vi "Maximize.vi"(8 "error in":errorcluster, 11 "Flex Subpanel in":refnum<class "Flex UI Subpanel.lvclass">) -> (0 "error out":errorcluster, 3 "Flex Subpanel out":refnum<class "Flex UI Subpanel.lvclass">)   [LabVIEW 2016, in "Flex UI Subpanel.lvclass"]
doc: "Maximizes the UI."
uses:
  Flex UI Subpanel.lvclass
  <vilib>/Utility/miscctls.llb/LVPositionTypeDef.ctl
  Flex UI Subpanel.lvclass/Flex UI Subpanel.ctl
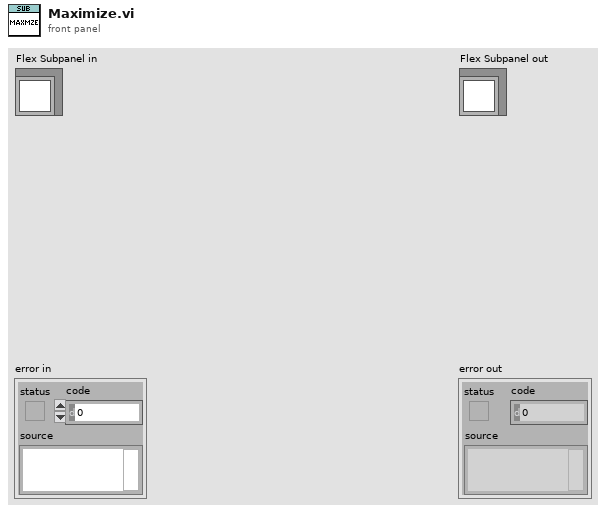
[diagram p1: front panel]
types:
  T1 = typedef "LVPositionTypeDef.ctl" = cluster{"Left":i32, "Top":i32}
  T2 = typedef "LVBoundsTypeDef.ctl" = cluster{"Width":u32, "Height":u32}
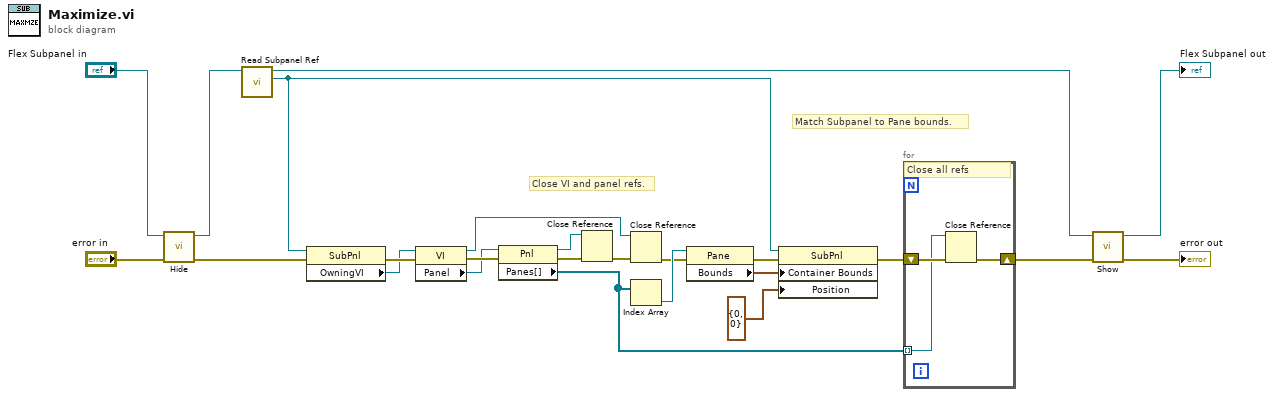
[diagram p0: block diagram]
diagram:
  # "Match Subpanel to Pane bounds."
  # "Close VI and panel refs."
  n1 = call-dynamic "Hide.vi"("error in"="error in", "Flex Subpanel in"="Flex Subpanel in") -> ("error out"=w4:errorcluster, "Flex Subpanel out"=w2:refnum<class "Flex UI Subpanel.lvclass">)  [unwired: 8 in]
  n2 = call "Read Subpanel Ref.vi"("Flex Subpanel in"=w2) -> ("Subpanel Ref"=w12:refnum<vi>, "Flex Subpanel out"=w20:refnum<class "Flex UI Subpanel.lvclass">)  [unwired: 9 in]
  n3 = property class="SubPnl"(reference=w12, error in=w4) -> (error out=w22:errorcluster, "OwningVI"=w18:refnum<vi>)  [unwired: 1 out]
  n4 = property class="VI"(reference=w18, error in=w22) -> (reference out=w8:refnum<vi>, error out=w24:errorcluster, "Panel"=w17:refnum<vi>)
  n5 = property class="Pnl"(reference=w17, error in=w24) -> (reference out=w11:refnum<vi>, error out=w15:errorcluster, "Panes[]"=w5:refnum<vi>[])
  n6 = Close Reference(reference=w11, error in (no error)=w15) -> (error out=w10:errorcluster)
  n7 = Close Reference(reference=w8, error in (no error)=w10) -> (error out=w9:errorcluster)
  n8 = Index Array(array=w5) -> (element=w14:refnum<vi>)  [unwired: 1 in]
  n9 = property on="MainPane" class="Pane"(reference=w14, error in=w9) -> (error out=w16:errorcluster, "Bounds"=w13:T2)  [unwired: 1 out]
  n10 = property on="Inactive SubPanel" class="SubPnl"(reference=w12, error in=w16, "Container Bounds"=w13, "Position"=T1 {"Left"=0, "Top"=0}) -> (error out=w6:errorcluster)  [unwired: 1 out]
  n11 = for {
    shift-right: [w26] -> w7
    shift-left: w6 -> [w27]
    tunnel: w5 -> [w25] mode=indexing
    # "Close all refs"
    n12 = Close Reference(reference=w25, error in (no error)=w27) -> (error out=w26:errorcluster)
  }
  n13 = call-dynamic "Show.vi"("error in"=w7, "Flex Subpanel in"=w20) -> ("error out"=→"error out":errorcluster, "Flex Subpanel out"=→"Flex Subpanel out":refnum<class "Flex UI Subpanel.lvclass">)  [unwired: 8 in]
